vi "Write Ext by Value.vi"(8 "Error In":errorcluster, 9 "Data":u8[](array[numeric]), 10 "Type":i8, 11 "Writer In":refnum<class "Writer.lvclass">) -> (0 "Error Out":errorcluster, 3 "Writer Out":refnum<class "Writer.lvclass">)   [LabVIEW 2018, in "Toolkit.lvlib" / "Writer.lvclass"]
uses:
  Writer.lvclass
  Writer.lvclass/Writer.ctl
  Public/Status/Read Is Error.vi
  Public/Status/Read Status.vi
  Public/Status/Read Status Message.vi
  Utility/Status Code.vi
  <vilib>/Utility/error.llb/Error Cluster From Error Code.vi
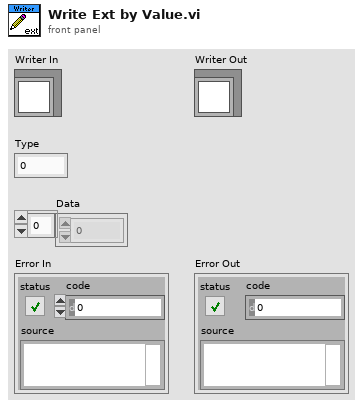
[diagram p1: front panel]
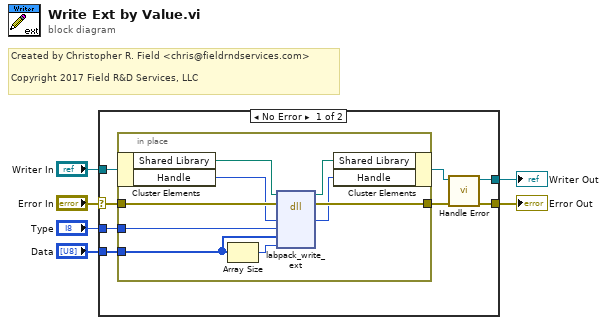
[diagram p0: block diagram]
diagram:
  # "Created by Christopher R. Field <chris@fieldrndservices.com>\n\nCopyright 2017 Field R&D Services, LLC"
  n1 = case shown="No Error" "Error In" {
    selector: "Error In" -> [w14 w24]
    tunnel: "Writer In" -> [w13 w25]
    tunnel: [w11 w25] -> w4
    tunnel: [w9 w24] -> w3
    tunnel: "Data" -> [w8 _]
    tunnel: "Type" -> [w7 _]
    frame No Error {
      n2 = in-place {
        in-place-border: w14 -> [w23]
        in-place-border: [w22] -> w10
        in-place-border: w8 -> [w17]
        in-place-border: w7 -> [w15]
        n3 = in-place-cluster #1(w13) -> ("Shared Library"=w19:path, "Handle"=w21:u64)
        n4 = Array Size(array=w17) -> (size(s)=w16:i32)
        n5 = dll-call lib="D:/Users/cfield/Code/MessagePack/LabPack/LabVIEW/trunk/src/LabPack/Private/labpack-x64.dll" fn="labpack_write_ext"(path in=w19, error in=w23, "writer"=w21, "type"=w15, "data"=w17, "count"=w16) -> (path out=w18:path, error out=w22:errorcluster, "writer"=w20:u64)  [unwired: 5 in]
        n6 = in-place-cluster #1("Shared Library"=w18, "Handle"=w20) -> (w12:refnum<class "Writer.lvclass">)
      }
      n7 = call "Handle Error.vi"("Error In"=w10, "Writer In"=w12) -> ("Error Out"=w9:errorcluster, "Writer Out"=w11:refnum<class "Writer.lvclass">)  [unwired: 8 in]
    }
    frame Error {
    }
  }
  "Writer Out" <- w4
  "Error Out" <- w3
